vi "Generate_Cage_DAQmx_Image_and_Scaling.vi"(7 "Draw Area Size":T4={"Width"=480, "Height"=480}, 8 "Error In":errorcluster, 9 "Target scale factor the max displayed cage size":dbl=0.96 format="%#_13g", 10 "Background color":u32(colorbox)=13816530, 11 "Cage Dims.":T2={"Width, mm"=180.0, "Height, mm"=180.0}) -> (0 "Error Out":errorcluster, 2 "Image Geometry and Scilng info":T1, 3 "Cage background Image":T3(plugin-control))   [LabVIEW 2018, in "Cage Diagram.lvlib"]
uses:
  Cage Diagram.lvlib
  SubVi's/Controls/CTL_Draw_Area_Size.ctl
  Typedefs/CTL_Cage_dimensions.ctl
  Typedefs/CTL_Image_Geomety_and_Scaling_info.ctl
  Common_Resources.lvlib
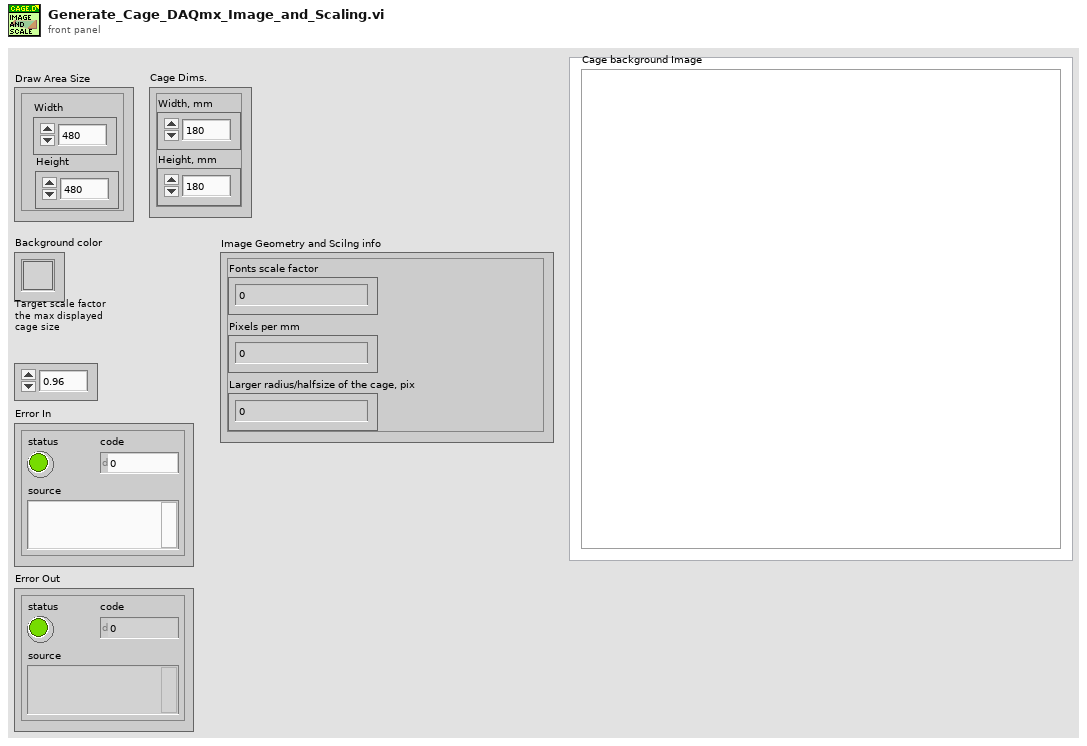
[diagram p1: front panel]
types:
  T1 = typedef "Cage Diagram.lvlib/CTL_Image_Geomety_and_Scaling_info.ctl" = cluster{"Fonts scale factor":dbl, "Pixels per mm":dbl, "Larger radius/halfsize of the cage, pix":dbl}
  T2 = typedef "Cage Diagram.lvlib/CTL_Cage_dimensions.ctl" = cluster{"Width, mm":dbl, "Height, mm":dbl}
  T3 = typedef "IMAQ Image.ctl" = refnum<image>
  T4 = typedef "Common_Resources.lvlib/CTL_Draw_Area_Size.ctl" = cluster{"Width":i32, "Height":i32}
  T5 = cluster{"Left":i32, "Top":i32, "Right":i32, "Bottom":i32}
  T6 = typedef "Image Type" = u32
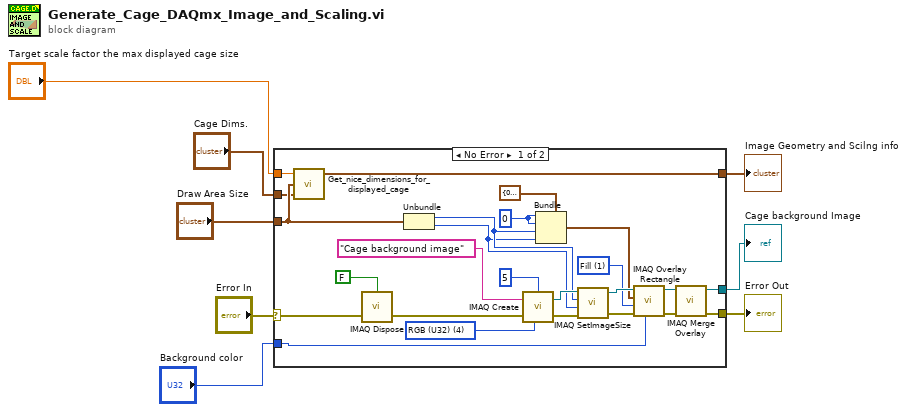
[diagram p0: block diagram]
diagram:
  n1 = case shown="No Error" "Error In" {
    selector: "Error In" -> [w9 w34]
    tunnel: "Target scale factor the max displayed cage size" -> [w33 _]
    tunnel: [w17 w34] -> w7
    tunnel: [w16 _] -> w6
    tunnel: "Background color" -> [w15 _]
    tunnel: "Draw Area Size" -> [w12 _]
    tunnel: "Cage Dims." -> [w11 _]
    tunnel: [w10 _] -> w2
    frame No Error {
      w20 = 0 ("Left")
      w25 = u32 1 items=["Frame", "Fill", "Highlight"] ("Drawing Mode (Frame)")
      w30 = T6 4 items=["Grayscale (U8)", "Grayscale (I16)", "Grayscale (SGL)", "Complex (CSG)", "RGB (U32)", "HSL (U32)", "RGB (U64)", "Grayscale (U16)"] ("Image Type")
      n2 = call "Get_nice_dimensions_for_displayed_cage.vi"("Cage Dims."=w11, "Draw Area Size"=w12, "Target scale factor the max displayed cage size"=w33) -> ("Image Geometry and Scilng info"=w10:T1)  [unwired: 2 in]
      n3 = call "IMAQ Dispose"("All Images? (No)"=FALSE, "error in (no error)"=w9) -> ("error out"=w14:errorcluster)  [unwired: 4 in]
      n4 = Unbundle(w12) -> ("Width"=w22:i32, "Height"=w21:i32)
      n5 = call "IMAQ Create"("Border Size"=5, "Image Name"="Cage background image", "Image Type"=w30, "error in (no error)"=w14) -> ("New Image"=w28:T3, "error out"=w29:errorcluster)  [unwired: 1 in]
      n6 = Bundle(cluster=T5 {"Left"=0, "Top"=0, "Right"=480, "Bottom"=480} ("Rectangle"), "Left"=w20, "Top"=w20, "Right"=w22, "Bottom"=w21) -> (w23:T5)
      n7 = call "IMAQ SetImageSize"("error in (no error)"=w29, "Y Resolution"=w21, "X Resolution"=w22, "Image"=w28) -> ("error out"=w27:errorcluster, "Image Out"=w26:T3)  [unwired: 1 in]
      n8 = call "IMAQ Overlay Rectangle"("Color"=w15, "error in (no error)"=w27, "Drawing Mode (Frame)"=w25, "Rectangle"=w23, "Image"=w26) -> ("error out"=w18:errorcluster, "Image Out"=w19:T3)  [unwired: 5 in]
      n9 = call "IMAQ Merge Overlay"("error in (no error)"=w18, "Image Src"=w19) -> ("error out"=w17:errorcluster, "Image Dst Out"=w16:T3)  [unwired: 8 in]
    }
    frame Error {
    }
  }
  "Error Out" <- w7
  "Cage background Image" <- w6
  "Image Geometry and Scilng info" <- w2
